vi "add log.vi"(8 "error in (ignored)":errorcluster, 10 "text":string) -> (0 "error dup":errorcluster)   [LabVIEW 2020]
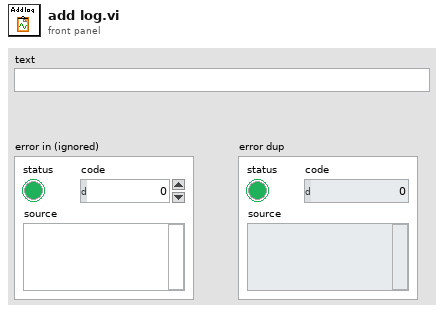
[diagram p1: front panel]
types:
  T1 = enum16{"open", "replace", "create", "open or create", "replace or create", "replace or create with confirmation"}
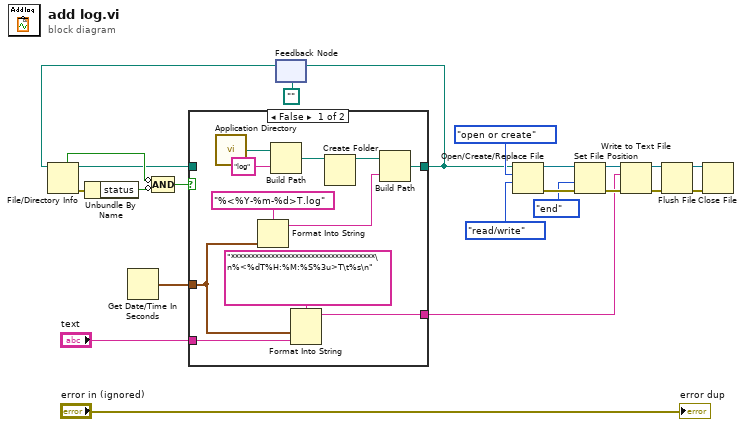
[diagram p0: block diagram]
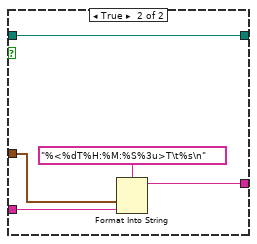
[diagram p2: hidden frame]
diagram:
  n1 = Get Date/Time In Seconds() -> (seconds since 1Jan1904=w3:timestamp)
  n2 = feedback #1(path "") -> (w21:path)
  n3 = File/Directory Info(path=w21) -> (path out=w16:path, directory=w20:bool, error out=w18:errorcluster)  [unwired: 1 in, 4 out]
  n4 = Unbundle By Name(w18) -> ("status"=w17:bool)
  n5 = Compound Arithmetic op=AND(invert w20, invert w17) -> (w19:bool)
  n6 = case shown="False" w19 {
    tunnel: [w31 w39] -> w22
    tunnel: w16 -> [_ w39]
    tunnel: w3 -> [w26 w35]
    tunnel: "text" -> [w25 w37]
    tunnel: [w24 w36] -> w1
    frame False {
      n7 = call <vilib>:"Application Directory.vi"() -> ("Application Directory"=w28:path)
      n8 = Format Into String(format string="%<%Y-%m-%d>T.log", w26) -> (resulting string=w32:string)  [unwired: 2 in, 1 out]
      n9 = Build Path(base path=w28, name or relative path="log") -> (appended path=w29:path)
      n10 = Format Into String(format string="************************************\n%<%dT%H:%M:%S%3u>T\t%s\n", w26, w25) -> (resulting string=w24:string)  [unwired: 2 in, 1 out]
      n11 = Create Folder(path (use dialog)=w29) -> (created path=w34:path)  [unwired: 2 in, 2 out]
      n12 = Build Path(base path=w34, name or relative path=w32) -> (appended path=w31:path)
    }
    frame True {
      n13 = Format Into String(format string="%<%dT%H:%M:%S%3u>T\t%s\n", w35, w37) -> (resulting string=w36:string)  [unwired: 2 in, 1 out]
    }
  }
  n14 = feedback-in #1(w22) -> ()
  n15 = Open/Create/Replace File(file path (use dialog)=w22, operation (0:open)=T1."open or create", access (0:read/write)=enum16{"read/write", "read-only", "write-only"}."read/write") -> (refnum out=w9:refnum<file>, error out=w6:errorcluster)  [unwired: 3 in, 1 out]
  n16 = Set File Position(refnum=w9, from (0:start)=enum16{"start", "end", "current"}."end", error in=w6) -> (refnum out=w8:refnum<file>, error out=w7:errorcluster)  [unwired: 1 in]
  n17 = Write to Text File(file (use dialog)=w8, text=w1, error in=w7) -> (refnum out=w13:refnum<file>, error out=w14:errorcluster)  [unwired: 1 in, 1 out]
  n18 = Flush File(refnum=w13, error in=w14) -> (refnum out=w11:refnum<file>, error out=w12:errorcluster)
  n19 = Close File(refnum=w11, error in=w12) -> ()  [unwired: 2 out]
  "error dup" <- "error in (ignored)"
